vi "Parse EscapedVariable-Text.vi"(8 "Error In":errorcluster) -> (0 "Error Out":errorcluster)   [LabVIEW 2018, in "Tests.lvlib" / "Parser.lvlib"]
uses:
  Parser.lvlib
  src/Toolkit/Tokens/Text/Text.lvclass
  src/Toolkit/Tokens/EscapedVariable/EscapedVariable.lvclass
  src/Toolkit/Tokens/Keyable/API/Keyable.lvclass/Keyable.ctl
  src/Toolkit/Tokens/Keyable/API/Read Key.vi
  src/Toolkit/Readers/String/String.lvclass
  D:/Users/cfield/Code/Field R&D Services/Mustache/trunk/src/Toolkit/Readers/Abstract/Abstract.lvclass
  <vilib>/Utility/LVClass/Get LV Class Name.vi
  src/Toolkit/Tokens/Text/API/Read Content.vi
  <vilib>/addons/_JKI Toolkits/Caraya/classes/Assert/Assert Equal_Variant.vi
  src/Toolkit/Tokens/Keyable/API/Keyable.lvclass
  <vilib>/addons/_JKI Toolkits/Caraya/classes/Test/Test.lvclass
  src/Toolkit/Parser/Parser.lvclass
  <vilib>/addons/_JKI Toolkits/Caraya/classes/Assert/Assert.lvclass
  Tests.lvlib
  src/Toolkit/Tokens/Abstract/Abstract.lvclass
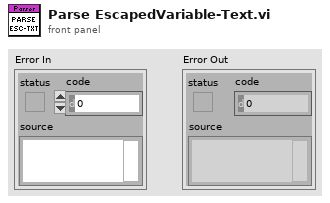
[diagram p1: front panel]
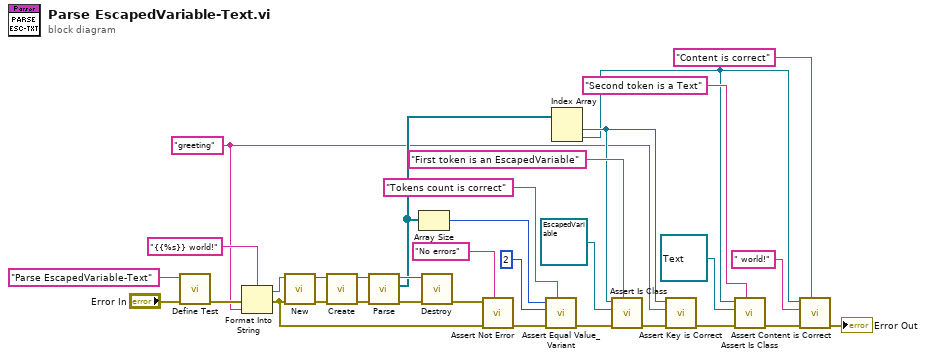
[diagram p0: block diagram]
diagram:
  w3 = "greeting" ("String")
  n1 = call <vilib>:"Define Test.vi"("error in (no error)"="Error In", "Label (VI Title)"="Parse EscapedVariable-Text") -> ("error out"=w24:errorcluster)  [unwired: 9 in]
  n2 = Format Into String(format string="{{%s}} world!", error in=w24, w3) -> (resulting string=w11:string, error out=w13:errorcluster)  [unwired: 1 in]
  n3 = call "New.vi"("Error In"=w13, "String"=w11) -> ("Error Out"=w30:errorcluster, "String"=w31:refnum<class "String.lvclass">)  [unwired: 8 in]
  n4 = call "Create.vi"("Error In"=w30, "Reader"=w31) -> ("Error Out"=w29:errorcluster, "Parser"=w28:refnum<class "Parser.lvclass">)  [unwired: 8 in]
  n5 = call "Parse.vi"("Error In"=w29, "Parser In"=w28) -> ("Error Out"=w26:errorcluster, "Tokens"=w18:refnum<class "Abstract.lvclass">[], "Parser Out"=w27:refnum<class "Parser.lvclass">)  [unwired: 7 in]
  n6 = Array Size(array=w18) -> (size(s)=w20:i32)
  n7 = call "Destroy.vi"("Error In"=w26, "Parser"=w27) -> ("Error Out"=w25:errorcluster)  [unwired: 9 in]
  n8 = call <vilib>:"Assert Not Error.vi"("Label"="No errors", "error in (no error)"=w13, "Not Error?"=w25) -> ("error out"=w22:errorcluster)  [unwired: 8 in]
  n9 = call <vilib>:"Assert Equal Value_Variant.vi"("Label"="Tokens count is correct", "error in (no error)"=w22, "Y"=2 ("size(s)"), "X"=w20) -> ("error out"=w8:errorcluster)  [unwired: 7 in]
  n10 = Index Array(array=w18) -> (element #1=w4:refnum<class "Abstract.lvclass">, element #2=w1:refnum<class "Abstract.lvclass">)  [unwired: 2 in]
  n11 = call "Assert Is Class.vi"("Label"="First token is an EscapedVariable", "Error In"=w8, "Expected"=refnum<class "EscapedVariable.lvclass"> refnum ("Mustache.lvlib:Tokens.lvlib:EscapedVariable.lvclass"), "Actual"=w4) -> ("Error Out"=w16:errorcluster)  [unwired: 7 in]
  n12 = call "Assert Key is Correct.vi"("Error In"=w16, "Expected"=w3, "Token"=w4) -> ("Error Out"=w6:errorcluster)  [unwired: 8 in]
  n13 = call "Assert Is Class.vi"("Label"="Second token is a Text", "Error In"=w6, "Expected"=refnum<class "Text.lvclass"> refnum ("Mustache.lvlib:Tokens.lvlib:Text.lvclass"), "Actual"=w1) -> ("Error Out"=w14:errorcluster)  [unwired: 7 in]
  n14 = call "Assert Content is Correct.vi"("Label"="Content is correct", "Error In"=w14, "Expected"=" world!", "Token"=w1) -> ("Error Out"=→"Error Out":errorcluster)  [unwired: 7 in]
